vi "Destroy Lookup.vi"(8 "error in (no error)":errorcluster, 11 "Lookup Service in":refnum<data-value>) -> (0 "error out":errorcluster, 1 "remaining references":refnum<data-value>[](array[refnum]))   [LabVIEW 2019, in "Lookup API.lvlib" / "Lookup Service.lvclass"]
doc: "<b>Description</b> Destroys and releases resources allocated by the Lookup. References to objects stored in the Lookup are also released.\n\n<b>Outputs</b>\n<b>remaining references</b>: References to all objects that had previously been registered in the Lookup.\n\nBSD 3-Clause License\n\nCopyright (c) 2021, TauTerra, LLC\nAll rights reserved.\n\nRedistribution and use in source and binary forms, with or without\nmodification, are permitted provided that the following conditions are met:\n\n1. Redistributions of source code must retain the above copyright notice, this\n list of conditions and the following disclaimer.\n\n2. Redistributions in binary form must reproduce the above copyright notice,\n this list of conditions and the following disclaimer in the documentation\n and/or other materials provided with the distribution.\n\n3. Neither the name of the copyright holder nor the names of its\n contributors may be used to endorse or promote products derived from\n this software without specific prior written permission.\n\nTHIS SOFTWARE IS PROVIDED BY THE COPYRIGHT HOLDERS AND CONTRIBUTORS \"AS IS\"\nAND ANY EXPRESS OR IMPLIED WARRANTIES, INCLUDING, BUT NOT LIMITED TO, THE\nIMPLIED WARRANTIES OF MERCHANTABILITY AND FITNESS FOR A PARTICULAR PURPOSE ARE\nDISCLAIMED. IN NO EVENT SHALL THE COPYRIGHT HOLDER OR CONTRIBUTORS BE LIABLE\nFOR ANY DIRECT, INDIRECT, INCIDENTAL, SPECIAL, EXEMPLARY, OR CONSEQUENTIAL\nDAMAGES (INCLUDING, BUT NOT LIMITED TO, PROCUREMENT OF SUBSTITUTE GOODS OR\nSERVICES; LOSS OF USE, DATA, OR PROFITS; OR BUSINESS INTERRUPTION) HOWEVER\nCAUSED AND ON ANY THEORY OF LIABILITY, WHETHER IN CONTRACT, STRICT LIABILITY,\nOR TORT (INCLUDING NEGLIGENCE OR OTHERWISE) ARISING IN ANY WAY OUT OF THE USE\nOF THIS SOFTWARE, EVEN IF ADVISED OF THE POSSIBILITY OF SUCH DAMAGE."
uses:
  Lookup Service.lvclass
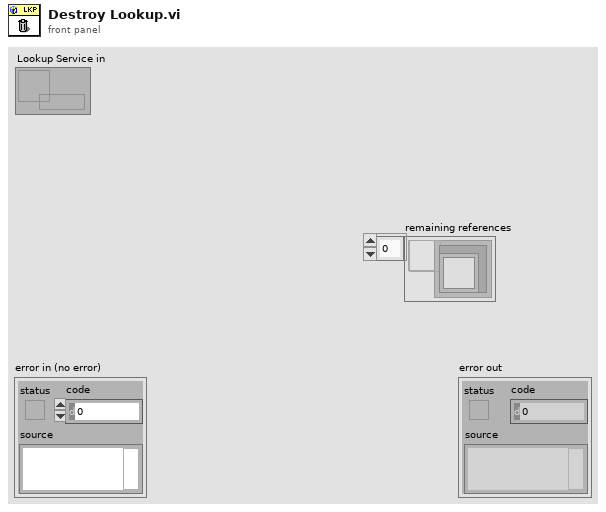
[diagram p1: front panel]
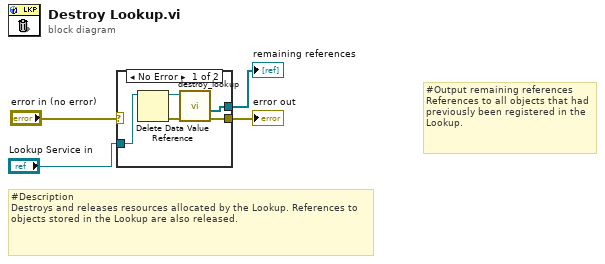
[diagram p0: block diagram]
diagram:
  # "#Output remaining references\nReferences to all objects that had previously been registered in the Lookup."
  # "#Description\nDestroys and releases resources allocated by the Lookup. References to objects stored in the Lookup are also released."
  n1 = case shown="No Error" "error in (no error)" {
    selector: "error in (no error)" -> [_ w10]
    tunnel: "Lookup Service in" -> [w9 _]
    tunnel: [w6 w10] -> w3
    tunnel: [w5 _] -> w1
    frame No Error {
      n2 = Delete Data Value Reference(data value reference=w9) -> (data value=w8:refnum<class "Lookup Service.lvclass">, error out=w7:errorcluster)  [unwired: 1 in]
      n3 = call-dynamic "destroy_lookup.vi"("error in (no error)"=w7, "Lookup Service in"=w8) -> ("error out"=w6:errorcluster, "remaining references"=w5:refnum<data-value>[])  [unwired: 8 in]
    }
    frame Error {
    }
  }
  "error out" <- w3
  "remaining references" <- w1
